vi "Update_1layer_Wx.vi"(1 "Learning rate":dbl, 2 "1layer_Out_hx":dbl, 3 "Array_Weights_hx":dbl[](array[numeric]), 4 "Array_Inputs":dbl[](array[numeric]), 5 "Array_2layer_Weights_at_Index_hx":dbl[](array[numeric]), 6 "Array_Out_ox":dbl[](array[numeric]), 7 "Array_target_ox":dbl[](array[numeric])) -> (0 "Array_Weights_hx_updated":dbl[](array[numeric]))   [LabVIEW 2016]
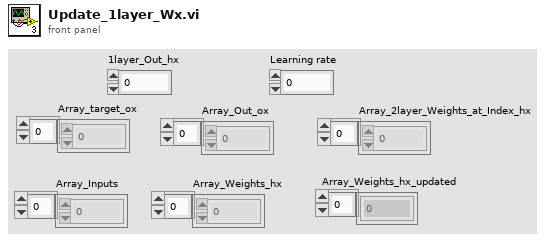
[diagram p1: front panel]
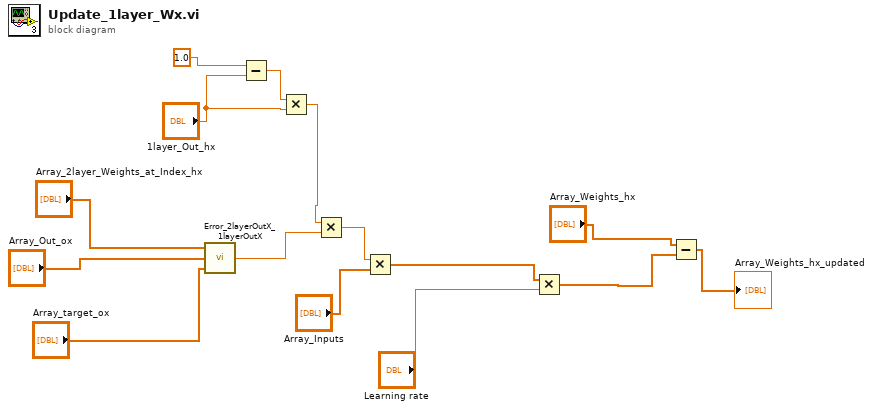
[diagram p0: block diagram]
diagram:
  n1 = call "Error_2layerOutX_1layerOutX.vi"("Array_target_ox"="Array_target_ox", "Array_Out_ox"="Array_Out_ox", "Array_2layer_Weights_at_Index_hx"="Array_2layer_Weights_at_Index_hx") -> ("Err_outX"=w10:dbl)
  n2 = Subtract(x=1.0, y="1layer_Out_hx") -> (x-y=w3:dbl)
  n3 = Multiply(x=w3, y="1layer_Out_hx") -> (x*y=w1:dbl)
  n4 = Multiply(x=w1, y=w10) -> (x*y=w13:dbl)
  n5 = Multiply(x=w13, y="Array_Inputs") -> (x*y=w11:dbl[])
  n6 = Multiply(x=w11, y="Learning rate") -> (x*y=w5:dbl[])
  n7 = Subtract(x="Array_Weights_hx", y=w5) -> (x-y=→"Array_Weights_hx_updated":dbl[])
